vi "solar_voy Set Bits (HDR_LENGTH).vi"(9 "HDR":T1, 10 "TCP Data (No HDR_LENGTH)":string) -> (1 "HDR_ID":u16, 2 "TCP Data out":string)   [LabVIEW 2018]
doc: "This updates the 'HDR_LENGTH' item in the TCP Data string. The 'HDR_ID' is returned to for updating the last value before the TCP message is written."
uses:
  solar_voy_def/solar_voy_def_ctl ITEM TYPE.ctl
  type/solar_type Item Type.ctl
  solar_voy_def/solar_voy_def_ctl ITEM.ctl
  solar_voy_def/solar_voy_def_ctl HDR.ctl
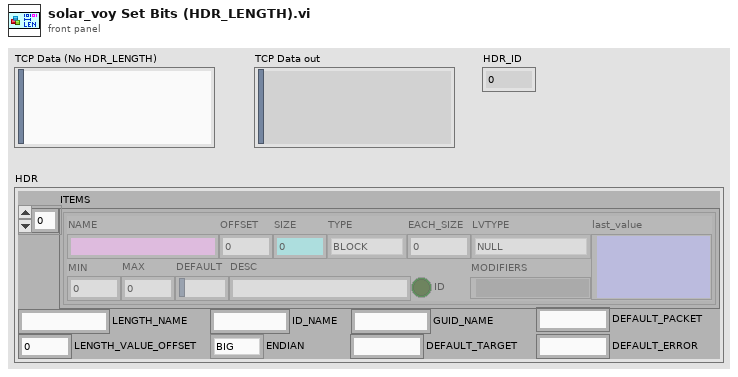
[diagram p1: front panel]
types:
  T1 = typedef "solar_voy_def_ctl HDR.ctl" = cluster{"ITEMS":T2[], "LENGTH_NAME":string, "LENGTH_VALUE_OFFSET":i32, "ID_NAME":string, "ENDIAN":enum8{"BIG", "LITTLE"}, "GUID_NAME":string, "DEFAULT_TARGET":string, "DEFAULT_PACKET":string, "DEFAULT_ERROR":string}
  T2 = typedef "solar_voy_def_ctl ITEM.ctl" = cluster{"NAME":string, "OFFSET":i32, "SIZE":i32, "TYPE":T3, "EACH_SIZE":i32, "LVTYPE":T4, "MIN":dbl, "MAX":dbl, "DEFAULT":string, "DESC":string, "ID":bool, "MODIFIERS":variant, "last_value":variant}
  T3 = typedef "solar_voy_def_ctl ITEM TYPE.ctl" = enum8{"BLOCK", "INT", "UINT", "FLOAT", "STRING"}
  T4 = typedef "solar_type Item Type.ctl" = enum16{"NULL", "UNKNOWN", "CLUSTER", "I8", "I16", "I32", "I64", "U8", "U16", "U32", "U64", "U8_ENUM", "U16_ENUM", "U32_ENUM", "SGL", "DBL", "BOOLEAN", "STRING", "PATH", "VISA", "TAG", "TIME", "I8_1D", "I16_1D", "I32_1D", "I64_1D", "U8_1D", "U16_1D", "U32_1D", "U64_1D", "U8_ENUM_1D", "U16_ENUM_1D", "U32_ENUM_1D", "SGL_1D", "DBL_1D", "BOOLEAN_1D", "STRING_1D", "PATH_1D", "VISA_1D", "TAG_1D", "TIME_1D", "I8_2D", "I16_2D", "I32_2D", "I64_2D", "U8_2D", "U16_2D", "U32_2D", "U64_2D", "U8_ENUM_2D", "U16_ENUM_2D", "U32_ENUM_2D", "SGL_2D", "DBL_2D", "BOOLEAN_2D", "STRING_2D", "PATH_2D", "VISA_2D", "TAG_2D", "TIME_2D"}
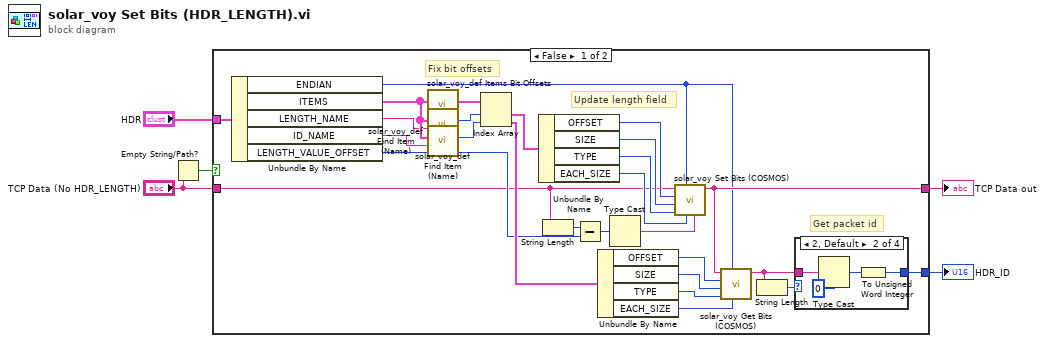
[diagram p0: block diagram]
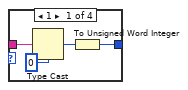
[diagram p2: hidden frame]
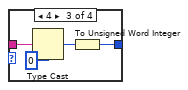
[diagram p3: hidden frame]
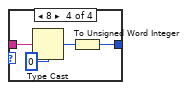
[diagram p4: hidden frame]
diagram:
  n1 = Empty String/Path?(string/path="TCP Data (No HDR_LENGTH)") -> (empty?=w1:bool)
  n2 = case shown="False" w1 {
    tunnel: [w32 _] -> w5
    tunnel: [w30 _] -> w4
    tunnel: "HDR" -> [w16 _]
    tunnel: "TCP Data (No HDR_LENGTH)" -> [w6 _]
    frame False {
      # "Get packet id"
      # "Fix bit offsets"
      # "Update length field"
      n3 = Unbundle By Name(w16) -> ("ENDIAN"=w31:enum8{"BIG", "LITTLE"}, "ITEMS"=w27:T2[], "LENGTH_NAME"=w9:string, "ID_NAME"=w26:string, "LENGTH_VALUE_OFFSET"=w8:i32)
      n4 = call "solar_voy_def Items Bit Offsets.vi"("ITEMS in"=w27) -> ("ITEMS with Bit Offsets"=w19:T2[])  [unwired: 9 in, 1 out]
      n5 = call "solar_voy_def Find Item (Name).vi"("ITEM_NAME"=w9, "ITEMS"=w27) -> ("Index"=w10:i32)  [unwired: 9 in]
      n6 = call "solar_voy_def Find Item (Name).vi"("ITEM_NAME"=w26, "ITEMS"=w27) -> ("Index"=w28:i32)  [unwired: 9 in]
      n7 = Index Array(array=w19, index #1=w10, index #2=w28) -> (element #1=w11:T2, element #2=w29:T2)
      n8 = Unbundle By Name(w11) -> ("OFFSET"=w12:i32, "SIZE"=w13:i32, "TYPE"=w17:T3, "EACH_SIZE"=w18:i32)
      n9 = String Length(string=w6) -> (length=w7:i32)
      n10 = Subtract(x=w7, y=w8) -> (x-y=w14:i32)
      n11 = Unbundle By Name(w29) -> ("OFFSET"=w24:i32, "SIZE"=w22:i32, "TYPE"=w23:T3, "EACH_SIZE"=w25:i32)
      n12 = Type Cast(x=w14) -> (*(type *) &x=w15:string)  [unwired: 1 in]
      n13 = call "solar_voy Set Bits (COSMOS).vi"("LabVIEW Flattened Value"=w15, "Bit Element Size (Array only)"=w18, "ENDIAN"=w31, "COSMOS TYPE"=w17, "Bit Size"=w13, "Bit Offset"=w12, "Padded COSMOS Data in"=w6) -> ("COSMOS Data out"=w32:string)  [unwired: 2 in, 2 out]
      n14 = call "solar_voy Get Bits (COSMOS).vi"("Bit Element Size (Array only)"=w25, "Endian (BIG)"=w31, "COSMOS TYPE"=w23, "Bit Size"=w22, "Bit Offset"=w24, "COSMOS Data"=w32) -> ("LabVIEW Flattened Value"=w20:string)  [unwired: 4 in, 1 out]
      n15 = String Length(string=w20) -> (length=w21:i32)
      n16 = case shown="2, Default" w21 {
        tunnel: w20 -> [w36 w40 w44 w48]
        tunnel: [w33 w37 w41 w45] -> w30
        frame 1 {
          n17 = Type Cast(type=u8 0, x=w36) -> (*(type *) &x=w34:u8)
          n18 = To Unsigned Word Integer(number=w34) -> (unsigned 16bit integer=w33:u16)
        }
        frame 2, Default {
          n19 = Type Cast(type=u16 0, x=w40) -> (*(type *) &x=w38:u16)
          n20 = To Unsigned Word Integer(number=w38) -> (unsigned 16bit integer=w37:u16)
        }
        frame 4 {
          n21 = Type Cast(type=u32 0, x=w44) -> (*(type *) &x=w42:u32)
          n22 = To Unsigned Word Integer(number=w42) -> (unsigned 16bit integer=w41:u16)
        }
        frame 8 {
          n23 = Type Cast(type=u64 0, x=w48) -> (*(type *) &x=w46:u64)
          n24 = To Unsigned Word Integer(number=w46) -> (unsigned 16bit integer=w45:u16)
        }
      }
    }
    frame True {
    }
  }
  "TCP Data out" <- w5
  "HDR_ID" <- w4
